vi "Ran.vi"(3 "offset":dbl(knob) scale=0.0..10.0 scale format="%.1f", 5 "mul fatt":dbl format="%.2f") -> (1 "out num":dbl format="%.2f")   [LabVIEW 2012]
doc: "Generatore random modificato"
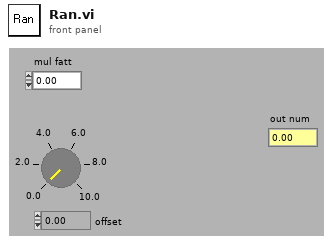
[diagram p1: front panel]
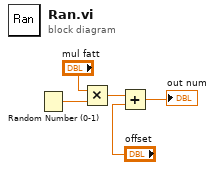
[diagram p0: block diagram]
diagram:
  n1 = Random Number (0-1)() -> (number: 0 to 1=w4:dbl)
  n2 = Multiply(x="mul fatt", y=w4) -> (x*y=w3:dbl)
  n3 = Add(x=w3, y="offset") -> (x+y=→"out num":dbl)
